vi "Stop Points.vi"(8 "error in":errorcluster, 11 "Sample PID Flow in":refnum<class "Sample PID Flow.lvclass">) -> (0 "error out":errorcluster, 3 "Sample PID Flow out":refnum<class "Sample PID Flow.lvclass">)   [LabVIEW 2023, in "Sample PID Flow.lvclass"]
uses:
  Sample PID Flow.lvclass
  Task/Task Base/Task Base.lvclass/Task Base.ctl
  Sample PID Flow.lvclass/Sample PID Flow.ctl
  Measure and Stimulus Subsystems/Measure and Stimulus Subsystems.lvclass
  Task/Task Base/Task Base.lvclass
  D:/git/HAL/HAL GOOP4/Task/Task Base/Task Base.lvclass
  D:/git/HAL/HAL GOOP4/Tests/Sample Tasks/Sample PID Flow/Sample PID Flow.lvclass
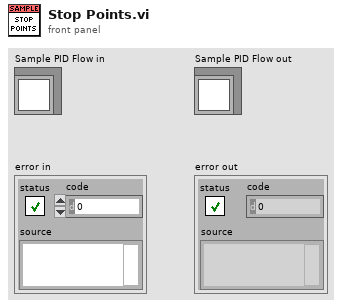
[diagram p1: front panel]
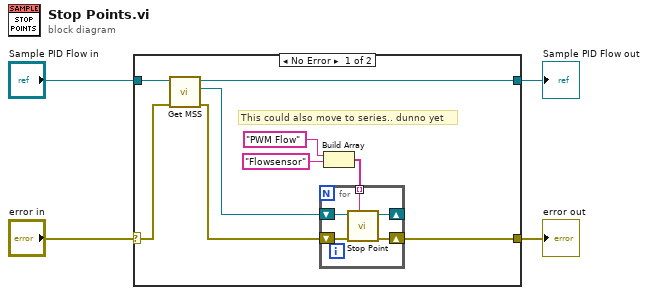
[diagram p0: block diagram]
diagram:
  n1 = case shown="No Error" "error in" {
    selector: "error in" -> [w8 w20]
    tunnel: [w5 w20] -> w3
    tunnel: [w9 w19] -> w1
    tunnel: "Sample PID Flow in" -> [w13 w19]
    frame No Error {
      # "This could also move to series.. dunno yet"
      n2 = call "Get MSS.vi"("error in (no error)"=w8, "Task Base in"=w13) -> ("error out"=w6:errorcluster, "MSS"=w7:refnum<class "Measure and Stimulus Subsystems.lvclass">, "Task Base out"=w9:refnum<class "Sample PID Flow.lvclass">)  [unwired: 7 in]
      n3 = Build Array("PWM Flow" ("Target Ident"), "Flowsensor" ("Target Identifier")) -> (w10:string[])
      n4 = for {
        shift-right: [w17] -> w5
        shift-left: w6 -> [w14]
        tunnel: w10 -> [w15] mode=indexing
        shift-right: [w16] -> _
        shift-left: w7 -> [w18]
        n5 = call "Stop Point.vi"("Point Ident"=w15, "error in"=w14, "MSS in"=w18) -> ("error out"=w17:errorcluster, "MSS out"=w16:refnum<class "Measure and Stimulus Subsystems.lvclass">)  [unwired: 7 in]
      }
    }
    frame Error {
    }
  }
  "error out" <- w3
  "Sample PID Flow out" <- w1
